vi "updateDataForStiffness.vi"(8 "error in (no error)":errorcluster, 11 "Model in":refnum<class "Model.lvclass">) -> (0 "error out":errorcluster, 3 "Model out":refnum<class "Model.lvclass">)   [LabVIEW 2015, in "Model.lvclass"]
uses:
  Model.lvclass
  Model.lvclass/Model.ctl
  <userlib>/Common/Devices/DistanceGauge/DistanceGauge/DistanceGauge.lvclass/DistanceGauge.ctl
  <userlib>/Common/Devices/ForceSensorCalculator/ForceSensorCalculator/ForceSensorCalculator.lvclass/ForceSensorCalculator.ctl
  ApplicationElements/StiffnessCalculator/StiffnessCalculator.lvclass
  <userlib>/Common/Devices/ForceSensorCalculator/ForceSensorCalculator/ForceSensorCalculator.lvclass
  <userlib>/Common/Devices/DistanceGauge/DistanceGauge/DistanceGauge.lvclass
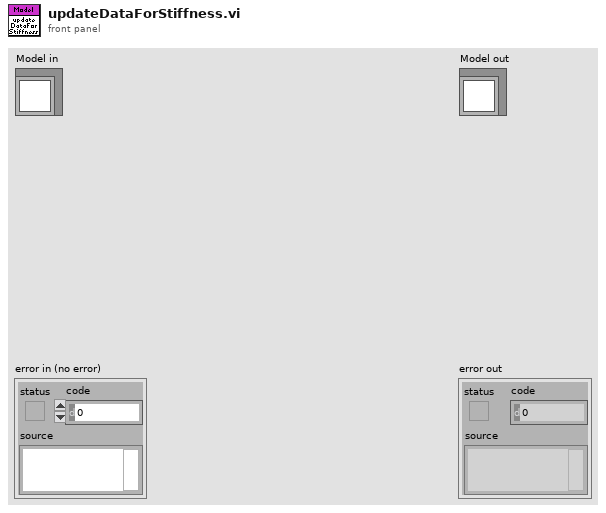
[diagram p1: front panel]
types:
  T1 = typedef "DistanceGauge.lvlib/Distance Data.ctl" = cluster{"Distance Measured 1":dbl[unit], "Distance Measured 2":dbl[unit]}
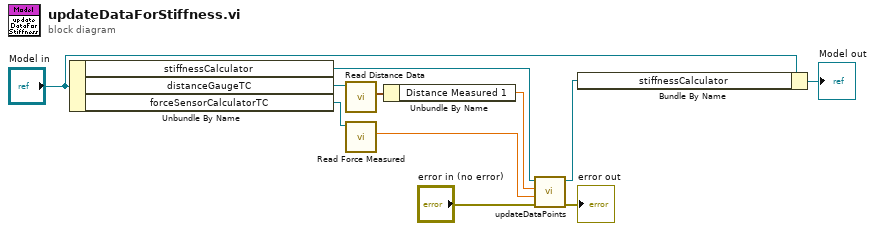
[diagram p0: block diagram]
diagram:
  n1 = Unbundle By Name("Model in") -> ("stiffnessCalculator"=w11:refnum<class "StiffnessCalculator.lvclass">, "distanceGaugeTC"=w5:refnum<class "DistanceGaugeTC.lvclass">, "forceSensorCalculatorTC"=w1:refnum<class "ForceSensorCalculatorTC.lvclass">)
  n2 = call <userlib>:"Read Distance Data.vi"("DistanceGauge in"=w5) -> ("Distance Data"=w4:T1)  [unwired: 9 in, 1 out]
  n3 = call <userlib>:"Read Force Measured.vi"("ForceSensor in"=w1) -> ("Force Demand"=w2:dbl[unit])  [unwired: 9 in, 1 out]
  n4 = Unbundle By Name(w4) -> ("Distance Measured 1"=w3:dbl[unit])
  n5 = call "updateDataPoints.vi"("error in (no error)"="error in (no error)", "Force Measured"=w2, "Distance Measured"=w3, "StiffnessCalculator in"=w11) -> ("error out"=→"error out":errorcluster, "StiffnessCalculator out"=w9:refnum<class "StiffnessCalculator.lvclass">)  [unwired: 6 in]
  n6 = Bundle By Name(cluster="Model in", "stiffnessCalculator"=w9) -> (→"Model out":refnum<class "Model.lvclass">)
